vi "userListView.vi"() -> ()   [LabVIEW 2019]
uses:
  03_Home/controller/logoutBtn.ctl
  03_Home/controller/exitBtn.ctl
  <vilib>/Utility/miscctls.llb/LVPointTypeDef.ctl
  03_Home/controller/pannelState.ctl
  globalValue.vi
panel:
  in  "backPage":bool
  out "totalCount":string
  in  "totalPage":i8
  in  "crrentPage":i8
  in  "leftBtn":bool
  in  "rightBtn":bool
  in  "btnGroup":T1
  out "userList":i32(listbox)
  in  "searchBtn":bool
  in  "searchForm":string
  in  "Help Button":bool
  in  "LogOut Button":T2
  in  "Exit Button":T3
  out "userNm":string
  # "/"
  # "|"
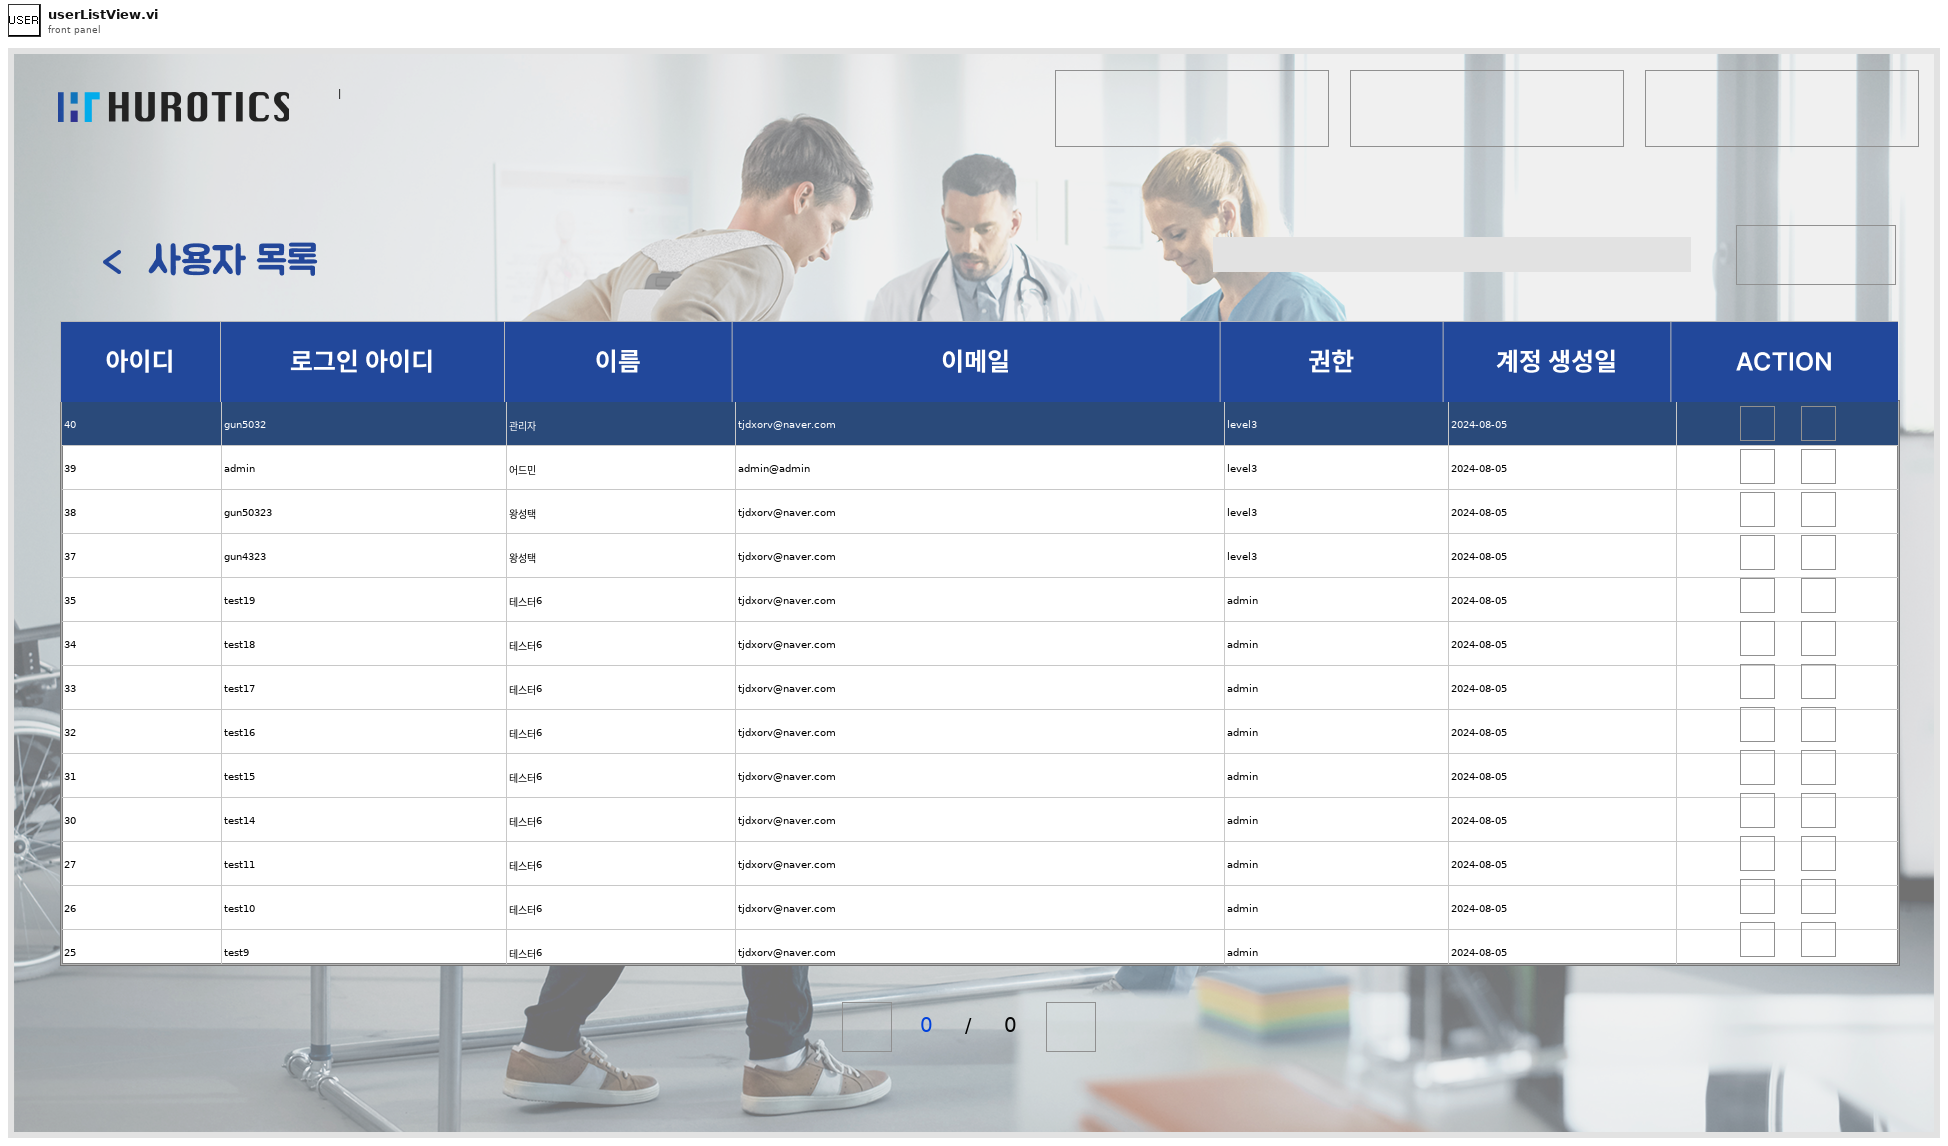
[diagram p1: front panel]
types:
  T1 = cluster{"updateBtn":bool, "deleteBtn":bool, "updateBtn 2":bool, "deleteBtn 2":bool, "updateBtn 3":bool, "deleteBtn 3":bool, "updateBtn 4":bool, "deleteBtn 4":bool, "updateBtn 5":bool, "deleteBtn 5":bool, "updateBtn 6":bool, "deleteBtn 6":bool, "updateBtn 7":bool, "deleteBtn 7":bool, "updateBtn 8":bool, "deleteBtn 8":bool, "updateBtn 9":bool, "deleteBtn 9":bool, "updateBtn 10":bool, "deleteBtn 10":bool, "updateBtn 11":bool, "deleteBtn 11":bool, "updateBtn 12":bool, "deleteBtn 12":bool, "updateBtn 13":bool, "deleteBtn 13":bool, "updateBtn 14":bool, "deleteBtn 14":bool, "updateBtn 15":bool, "deleteBtn 15":bool}
  T2 = typedef "logoutBtn.ctl" = bool
  T3 = typedef "exitBtn.ctl" = bool
  T4 = typedef "LVPointTypeDef.ctl" = cluster{"Horizontal":i16, "Vertical":i16}
  T5 = enum16{"connection", "create", "getReadList", "getRead", "getCount", "update", "delete", "close"}
  T6 = typedef "pannelState.ctl" = enum16{"Init", "LogIn", "SignUpView", "Home", "Management_patientList", "Management_patientTrashtList", "Management_patientCreate", "Management_patientUpdate", "Management_patientTraining", "Management_patientTrainingDetail", "H-MEDI PatientList", "H-MEDI HardwareCtl", "Adjust", "FineTuning", "UserList", "UserDetail", "Exit"}
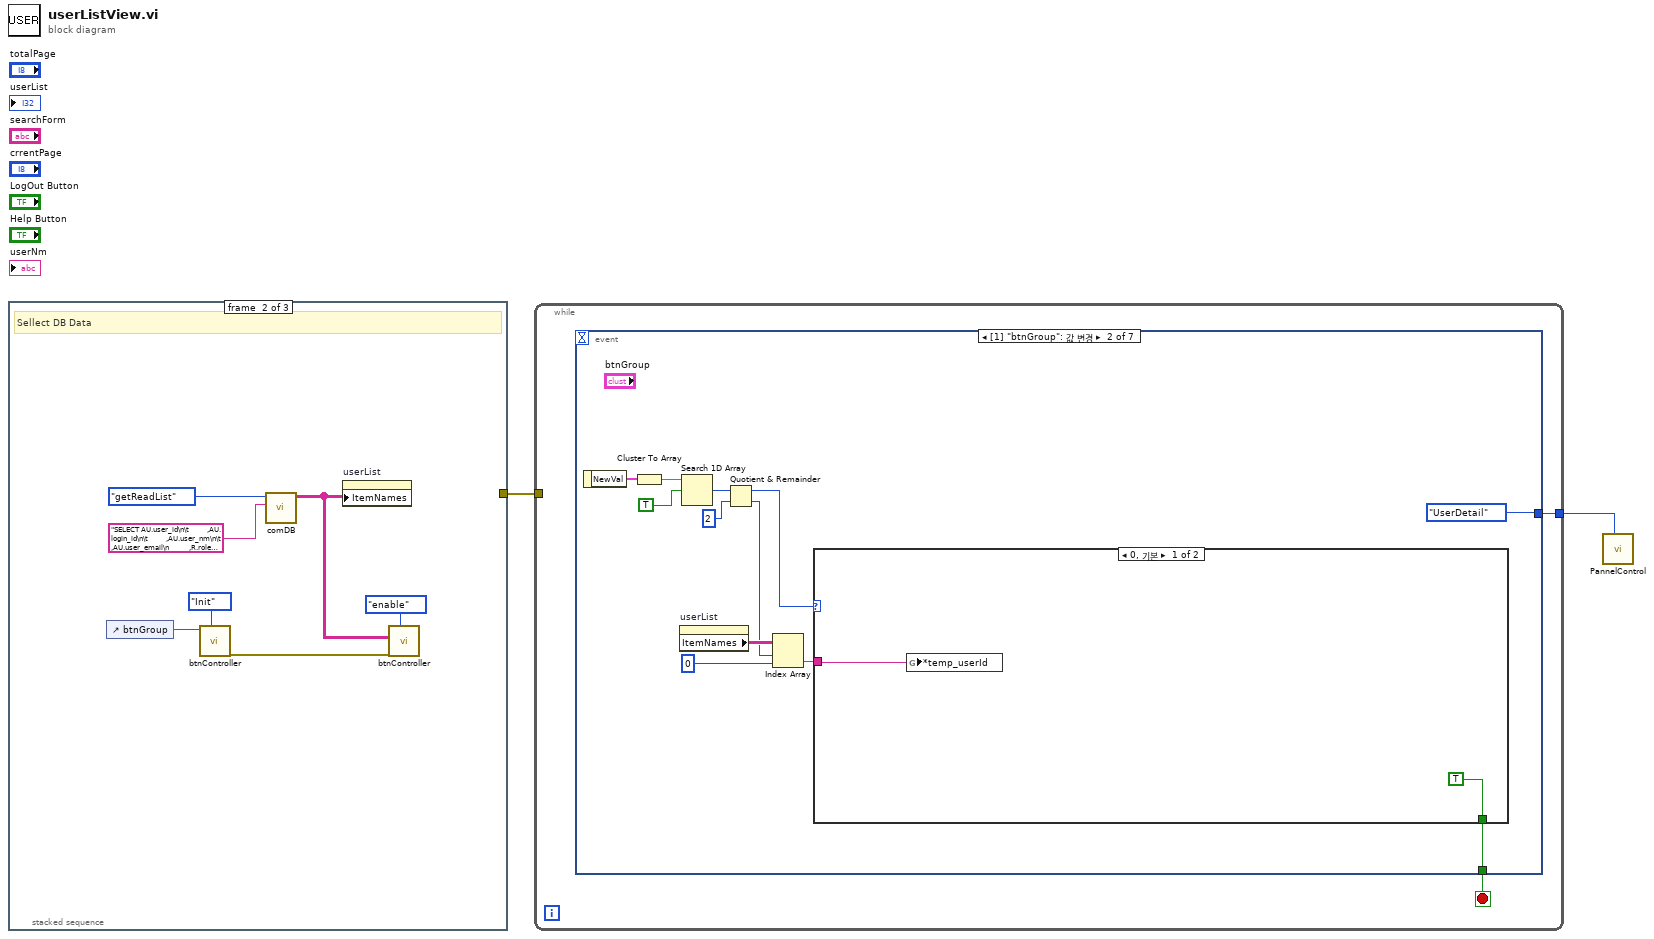
[diagram p0: block diagram]
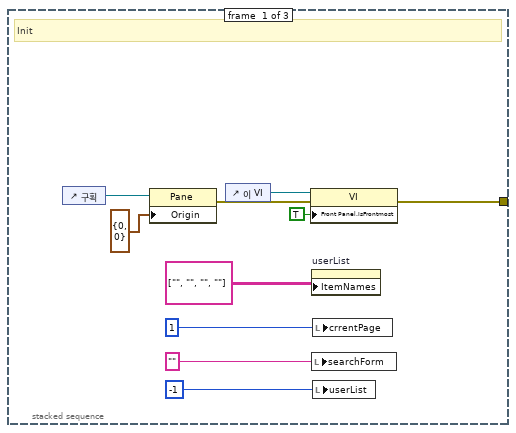
[diagram p2: hidden frame]
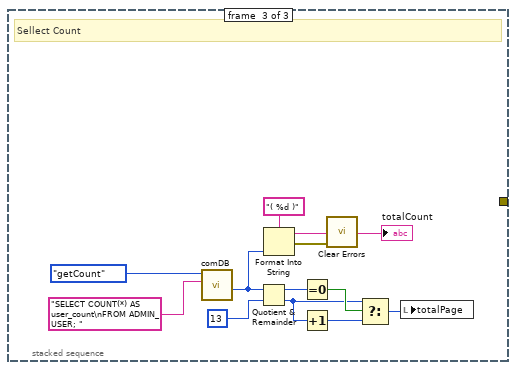
[diagram p3: hidden frame]
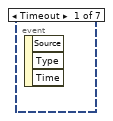
[diagram p4: hidden frame]
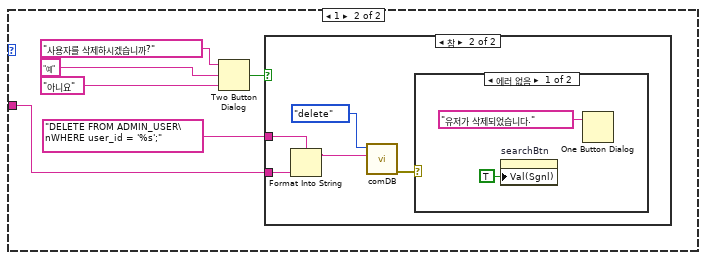
[diagram p5: hidden frame]
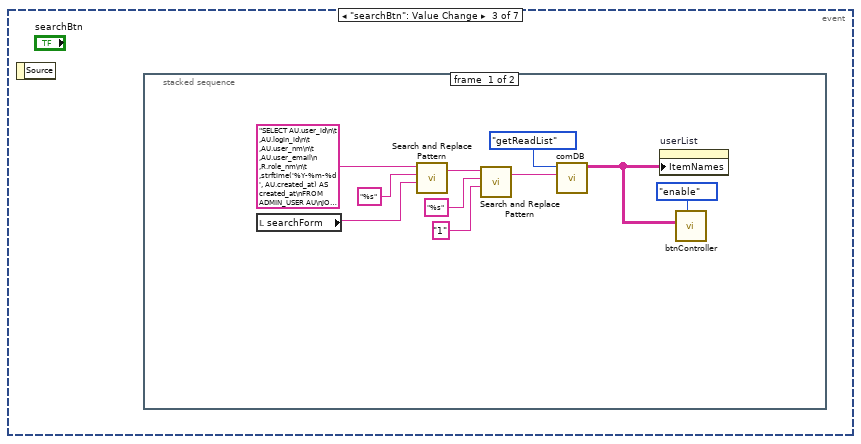
[diagram p8: hidden frame]
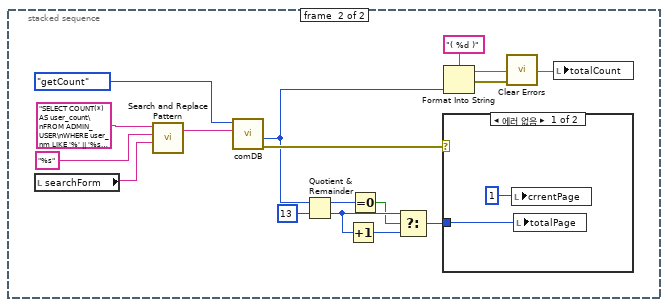
[diagram p9: hidden frame]
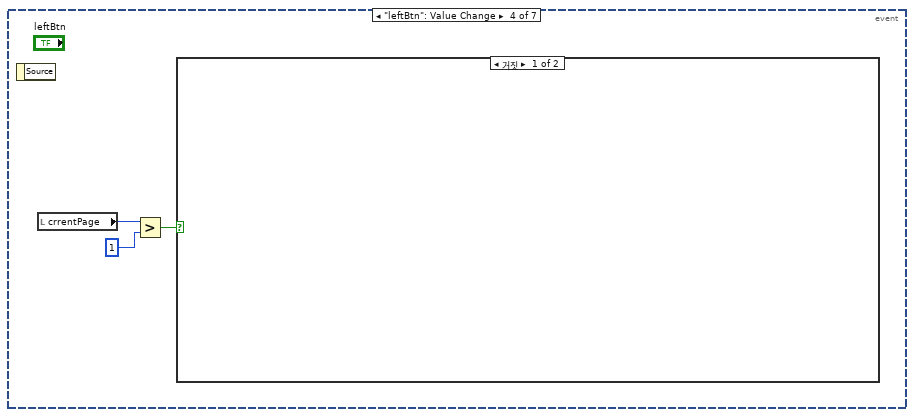
[diagram p11: hidden frame]
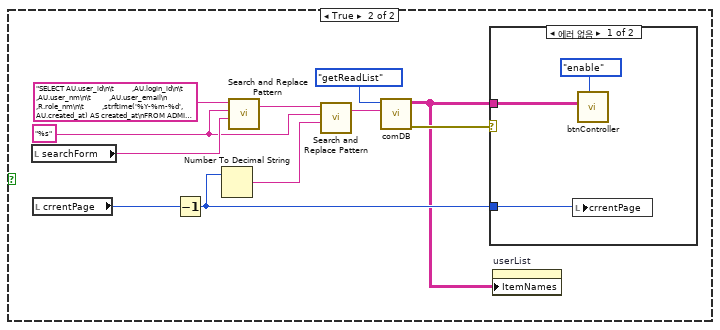
[diagram p12: hidden frame]
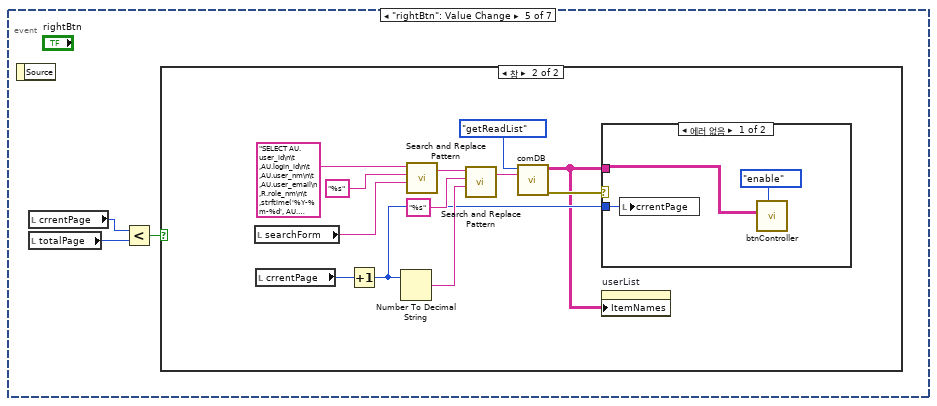
[diagram p14: hidden frame]
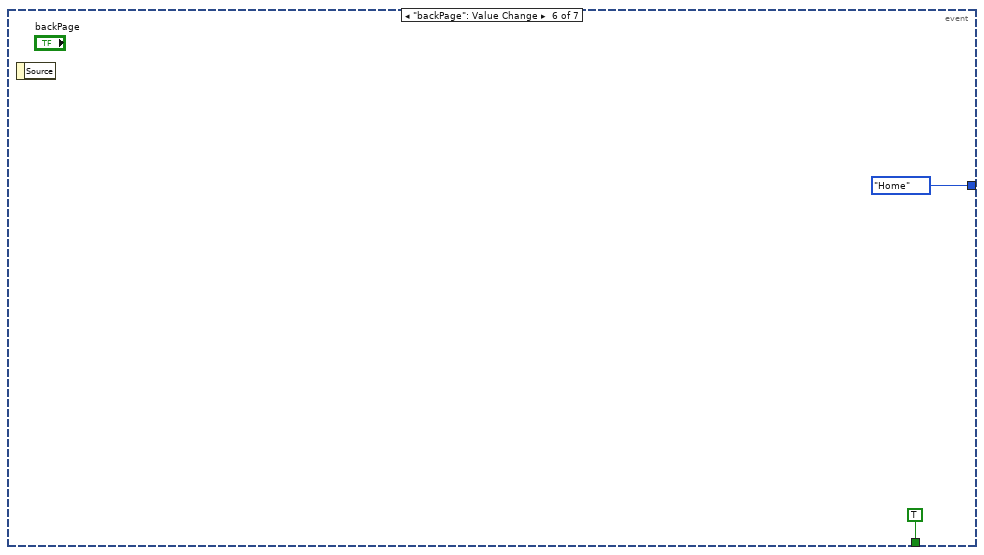
[diagram p17: hidden frame]
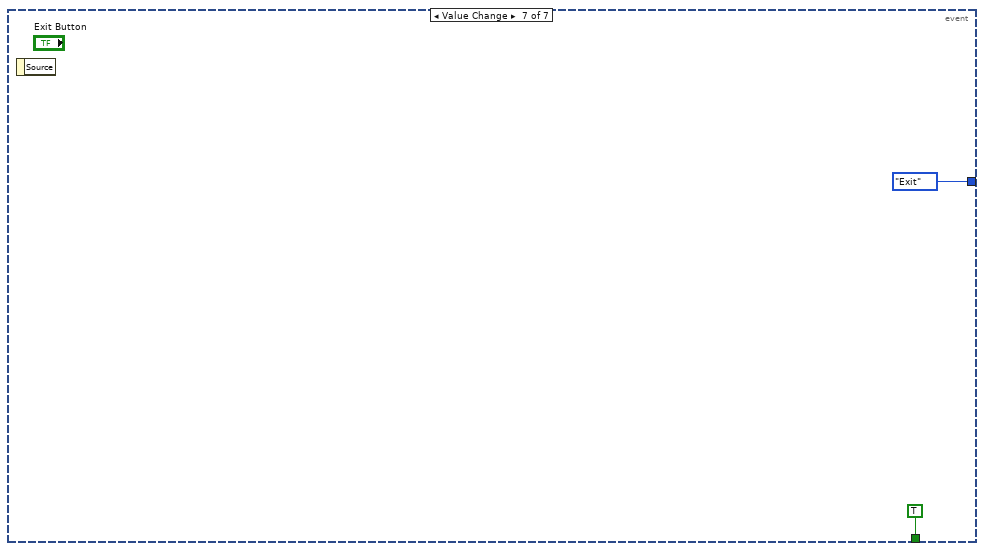
[diagram p18: hidden frame]
diagram:
  n1 = stacked-sequence {
    tunnel: [w3 _ _] -> w2
    frame #0 {
      # "Init"
      n2 = control-ref of="구획"() -> (w10:refnum<vi>)
      n3 = property class="Pane"(reference=w10, "Origin"=T4 {"Horizontal"=0, "Vertical"=0} ("원점")) -> (error out=w8:errorcluster)  [unwired: 1 in, 1 out]
      n4 = control-ref of="이 VI"() -> (w12:refnum<vi>)
      n5 = property class="VI"(reference=w12, error in=w8, "Front Panel.IsFrontmost"=TRUE ("프런트패널 윈도우:맨 앞으로")) -> (error out=w3:errorcluster)  [unwired: 1 out]
      n6 = property on="userList" class="MCListbox (엄격한)"("ItemNames"=string[][] [["", ""], ["", ""]]) -> ()  [unwired: 2 in, 2 out]
      n7 = local write "searchForm"("" ("searchForm")) -> ()
      n8 = local write "crrentPage"(i8 1 ("crrentPage")) -> ()
      n9 = local write "userList"(-1 ("userList")) -> ()
    }
    frame #1 {
      # "Sellect DB Data"
      n10 = control-ref of="btnGroup"() -> (w13:refnum<vi>)
      n11 = call "btnController.vi"("state"=enum16{"Init", "enable"}."Init", "btnGroup"=w13) -> ("error out"=w15:errorcluster)  [unwired: 9 in]
      n12 = call "comDB.vi"("Query"="SELECT AU.user_id\n\t         ,AU.login_id\n\t         ,AU.user_nm\n\t         ,AU.user_email\n          ,R.role_nm\n\t         ,strftime('%Y-%m-%d', AU.created_at) AS created_at\nFROM ADMIN_USER AU\nJOIN ROLE R ON AU.role_id = R.role_id\nWHERE AU.user_nm LIKE '%' || '' || '%'\nORDER BY AU.updated_at DESC \nLIMIT 13 OFFSET (1 - 1) * 13", "State"=T5."getReadList") -> ("resultList"=w17:string[][])  [unwired: 5 in, 3 out]
      n13 = property on="userList" class="MCListbox (엄격한)"("ItemNames"=w17) -> ()  [unwired: 2 in, 2 out]
      n14 = call "btnController.vi"("state"=enum16{"Init", "enable"}."enable", "error in (no error)"=w15, "2dArray"=w17) -> ()  [unwired: 8 in, 1 out]
    }
    frame #2 {
      # "Sellect Count"
      n15 = call "comDB.vi"("Query"="SELECT COUNT(*) AS user_count\nFROM ADMIN_USER; ", "State"=T5."getCount") -> ("count"=w23:i64)  [unwired: 5 in, 3 out]
      n16 = Quotient & Remainder(x=w23, y=i64 13) -> (x-y*floor(x/y)=w25:i64, floor(x/y)=w24:i64)
      n17 = Format Into String(format string="( %d )" ("포맷 문자열"), w23) -> (resulting string=→"totalCount":string, error out=w20:errorcluster)  [unwired: 2 in]
      n18 = Equal To 0?(x=w25) -> (x = 0?=w26:bool)
      n19 = Increment(x=w24) -> (x+1=w28:i64)
      n20 = call <vilib>:"Clear Errors.vi"("error in (no error)"=w20) -> ()  [unwired: 5 in, 2 out]
      n21 = Select(t=w24, s=w26, f=w28) -> (s? t:f=w27:i64)
      n22 = local write "totalPage"(w27) -> ()
    }
  }
  n23 = while {
    tunnel: w2 -> [_]
    tunnel: [w32] -> w1
    stop <- w33 stop-if-true
    n24 = event shown="[1] \"btnGroup\": 값 변경" {
      selector: _ -> [_ _ _ _ _ _ _]
      dyn-events: _ -> [_ _ _ _ _ _ _]
      timeout: _ -> [_ _ _ _ _ _ _]
      tunnel: [_ w35 _ _ _ TRUE TRUE] -> w33
      tunnel: [_ pannelState."UserDetail" ("State") _ _ _ pannelState."Home" ("State") pannelState."Exit" ("State")] -> w32
      event Timeout {
        n25 = event-data() -> ()  [unwired: 1 in, 3 out]
      }
      event "btnGroup": Value Change {
        n26 = event-data() -> ("NewVal"=w45:T1)  [unwired: 1 in]
        n27 = Cluster To Array(cluster=w45) -> (array=w44:bool[])
        n28 = property on="userList" class="MCListbox (엄격한)"() -> ("ItemNames"=w40:string[][])  [unwired: 2 in, 2 out]
        n29 = Search 1D Array(1D array=w44, element=TRUE ("원소")) -> (index of element=w42:i32)  [unwired: 1 in]
        n30 = Quotient & Remainder(x=w42, y=2) -> (x-y*floor(x/y)=w36:i32, floor(x/y)=w37:i32)
        n31 = Index Array(array=w40, index (row)=w37, index (col)=0 ("비활성화된 인덱스 (열)")) -> (element=w38:string)
        n32 = case shown="0, 기본" w36 {
          tunnel: w38 -> [w46 w48]
          tunnel: [TRUE _] -> w35
          frame 0, Default {
            n33 = global write "globalValue.vi" "*temp_userId"(w46) -> ()
          }
          frame 1 {
            n34 = Two Button Dialog(message="사용자를 삭제하시겠습니까?" ("메시지"), 1:"아니요" ("거짓 버튼 이름(\"취소\")"), 2:"예" ("참 버튼 이름(\"확인\")")) -> (T button?=w49:bool)
            n35 = case shown="참" w49 {
              tunnel: "DELETE FROM ADMIN_USER\nWHERE user_id = '%s';" ("Query") -> [_ w57]
              tunnel: w48 -> [_ w54]
              frame False {
              }
              frame True {
                n36 = Format Into String(format string=w57, w54) -> (resulting string=w56:string)  [unwired: 2 in, 1 out]
                n37 = call "comDB.vi"("Query"=w56, "State"=T5."delete") -> ("error out"=w55:errorcluster)  [unwired: 5 in, 3 out]
                n38 = case shown="에러 없음" w55 {
                  frame No Error {
                    n39 = property on="searchBtn" class="Bool (엄격한)"("Val(Sgnl)"=TRUE ("값(신호)")) -> ()  [unwired: 2 in, 2 out]
                    n40 = One Button Dialog(message="유저가 삭제되었습니다." ("메시지")) -> ()  [unwired: 1 in, 1 out]
                  }
                  frame Error {
                  }
                }
              }
            }
          }
        }
      }
      event "searchBtn": Value Change {
        n41 = event-data() -> ()  [unwired: 1 in, 1 out]
        n42 = stacked-sequence {
          frame #0 {
            n43 = local read "searchForm"() -> (w67:string)
            n44 = call <vilib>:"Search and Replace Pattern.vi"("string"="SELECT AU.user_id\n\t         ,AU.login_id\n\t         ,AU.user_nm\n\t         ,AU.user_email\n          ,R.role_nm\n\t         ,strftime('%Y-%m-%d', AU.created_at) AS created_at\nFROM ADMIN_USER AU\nJOIN ROLE R ON AU.role_id = R.role_id\nWHERE AU.user_nm LIKE '%' || '%s' || '%'\nORDER BY AU.updated_at DESC \nLIMIT 13 OFFSET (%s - 1) * 13" ("Query"), "regular expression (\"\")"="%s" ("regular expression (\"\")"), "replace string (\"\")"=w67) -> ("result string"=w66:string)  [unwired: 2 in, 1 out]
            n45 = call <vilib>:"Search and Replace Pattern.vi"("string"=w66, "regular expression (\"\")"="%s" ("regular expression (\"\")"), "replace string (\"\")"="1" ("regular expression (\"\")")) -> ("result string"=w63:string)  [unwired: 2 in, 1 out]
            n46 = call "comDB.vi"("Query"=w63, "State"=T5."getReadList") -> ("resultList"=w62:string[][])  [unwired: 5 in, 3 out]
            n47 = property on="userList" class="MCListbox (엄격한)"("ItemNames"=w62) -> ()  [unwired: 2 in, 2 out]
            n48 = call "btnController.vi"("state"=enum16{"Init", "enable"}."enable", "2dArray"=w62) -> ()  [unwired: 9 in, 1 out]
          }
          frame #1 {
            n49 = local read "searchForm"() -> (w86:string)
            n50 = call <vilib>:"Search and Replace Pattern.vi"("string"="SELECT COUNT(*) AS user_count\nFROM ADMIN_USER\nWHERE user_nm LIKE '%' || '%s' || '%'" ("Query"), "regular expression (\"\")"="%s" ("regular expression (\"\")"), "replace string (\"\")"=w86) -> ("result string"=w83:string)  [unwired: 2 in, 1 out]
            n51 = call "comDB.vi"("Query"=w83, "State"=T5."getCount") -> ("error out"=w82:errorcluster, "count"=w71:i64)  [unwired: 5 in, 2 out]
            n52 = Quotient & Remainder(x=w71, y=i64 13) -> (x-y*floor(x/y)=w76:i64, floor(x/y)=w77:i64)
            n53 = Increment(x=w77) -> (x+1=w79:i64)
            n54 = Equal To 0?(x=w76) -> (x = 0?=w75:bool)
            n55 = Select(t=w77, s=w75, f=w79) -> (s? t:f=w78:i64)
            n56 = case shown="에러 없음" w82 {
              tunnel: w78 -> [w87 _]
              frame No Error {
                n57 = local write "crrentPage"(i8 1 ("crrentPage")) -> ()
                n58 = local write "totalPage"(w87) -> ()
              }
              frame Error {
              }
            }
            n59 = Format Into String(format string="( %d )" ("포맷 문자열"), w71) -> (resulting string=w72:string, error out=w74:errorcluster)  [unwired: 2 in]
            n60 = call <vilib>:"Clear Errors.vi"("error in (no error)"=w74) -> ()  [unwired: 5 in, 2 out]
            n61 = local write "totalCount"(w72) -> ()
          }
        }
      }
      event "leftBtn": Value Change {
        n62 = event-data() -> ()  [unwired: 1 in, 1 out]
        n63 = local read "crrentPage"() -> (w89:i8)
        n64 = Greater?(x=w89, y=1) -> (0:w91:bool)
        n65 = case shown="거짓" w91 {
          frame False {
          }
          frame True {
            w92 = "%s" ("regular expression (\"\")")
            n66 = local read "searchForm"() -> (w96:string)
            n67 = local read "crrentPage"() -> (w102:i8)
            n68 = Decrement(x=w102) -> (x-1=w97:i8)
            n69 = Number To Decimal String(number=w97) -> (decimal integer string=w101:string)  [unwired: 1 in]
            n70 = call <vilib>:"Search and Replace Pattern.vi"("string"="SELECT AU.user_id\n\t         ,AU.login_id\n\t         ,AU.user_nm\n\t         ,AU.user_email\n          ,R.role_nm\n\t         ,strftime('%Y-%m-%d', AU.created_at) AS created_at\nFROM ADMIN_USER AU\nJOIN ROLE R ON AU.role_id = R.role_id\nWHERE AU.user_nm LIKE '%' || '%s' || '%'\nORDER BY AU.updated_at DESC \nLIMIT 13 OFFSET (%s - 1) * 13" ("Query"), "regular expression (\"\")"=w92, "replace string (\"\")"=w96) -> ("result string"=w94:string)  [unwired: 2 in, 1 out]
            n71 = call <vilib>:"Search and Replace Pattern.vi"("string"=w94, "regular expression (\"\")"=w92, "replace string (\"\")"=w101) -> ("result string"=w100:string)  [unwired: 2 in, 1 out]
            n72 = call "comDB.vi"("Query"=w100, "State"=T5."getReadList") -> ("error out"=w98:errorcluster, "resultList"=w93:string[][])  [unwired: 5 in, 2 out]
            n73 = case shown="에러 없음" w98 {
              tunnel: w97 -> [w105 _]
              tunnel: w93 -> [w104 _]
              frame No Error {
                n74 = local write "crrentPage"(w105) -> ()
                n75 = call "btnController.vi"("state"=enum16{"Init", "enable"}."enable", "2dArray"=w104) -> ()  [unwired: 9 in, 1 out]
              }
              frame Error {
              }
            }
            n76 = property on="userList" class="MCListbox (엄격한)"("ItemNames"=w93) -> ()  [unwired: 2 in, 2 out]
          }
        }
      }
      event "rightBtn": Value Change {
        n77 = event-data() -> ()  [unwired: 1 in, 1 out]
        n78 = local read "crrentPage"() -> (w107:i8)
        n79 = local read "totalPage"() -> (w106:i8)
        n80 = Less?(x=w107, y=w106) -> (x < y?=w108:bool)
        n81 = case shown="참" w108 {
          frame False {
          }
          frame True {
            n82 = local read "searchForm"() -> (w111:string)
            n83 = local read "crrentPage"() -> (w120:i8)
            n84 = Increment(x=w120) -> (x+1=w114:i8)
            n85 = Number To Decimal String(number=w114) -> (decimal integer string=w118:string)  [unwired: 1 in]
            n86 = call <vilib>:"Search and Replace Pattern.vi"("string"="SELECT AU.user_id\n\t         ,AU.login_id\n\t         ,AU.user_nm\n\t         ,AU.user_email\n          ,R.role_nm\n\t         ,strftime('%Y-%m-%d', AU.created_at) AS created_at\nFROM ADMIN_USER AU\nJOIN ROLE R ON AU.role_id = R.role_id\nWHERE AU.user_nm LIKE '%' || '%s' || '%'\nORDER BY AU.updated_at DESC \nLIMIT 13 OFFSET (%s - 1) * 13" ("Query"), "regular expression (\"\")"="%s" ("regular expression (\"\")"), "replace string (\"\")"=w111) -> ("result string"=w110:string)  [unwired: 2 in, 1 out]
            n87 = call <vilib>:"Search and Replace Pattern.vi"("string"=w110, "regular expression (\"\")"="%s" ("regular expression (\"\")"), "replace string (\"\")"=w118) -> ("result string"=w117:string)  [unwired: 2 in, 1 out]
            n88 = call "comDB.vi"("Query"=w117, "State"=T5."getReadList") -> ("error out"=w115:errorcluster, "resultList"=w109:string[][])  [unwired: 5 in, 2 out]
            n89 = case shown="에러 없음" w115 {
              tunnel: w114 -> [w123 _]
              tunnel: w109 -> [w122 _]
              frame No Error {
                n90 = local write "crrentPage"(w123) -> ()
                n91 = call "btnController.vi"("state"=enum16{"Init", "enable"}."enable", "2dArray"=w122) -> ()  [unwired: 9 in, 1 out]
              }
              frame Error {
              }
            }
            n92 = property on="userList" class="MCListbox (엄격한)"("ItemNames"=w109) -> ()  [unwired: 2 in, 2 out]
          }
        }
      }
      event "backPage": Value Change {
        n93 = event-data() -> ()  [unwired: 1 in, 1 out]
      }
      event Value Change {
        n94 = event-data() -> ()  [unwired: 1 in, 1 out]
      }
    }
  }
  n95 = call "PannelControl.vi"("State"=w1) -> ()  [unwired: 10 in, 1 out]
